vi "Generate Waveform in LV.vi"() -> (3 "a2":T1={"String"="This NULL (\u0000) is inside a LV Cluster", "Boolean"=FALSE, "Array"=[1.0+0.0i, 2.0+0.0i, 3.0+0.0i, 0.0+4.0i, 0.0+5.0i, 0.0+6.0i, 7.0+8.0i, 9.0+10.0i, -1.0-2.0i, -1e+20+1e+36i, 6.023e+23-1.23e-118i]}, 4 "waveform out":waveform(dbl), 6 "t0":timestamp, 8 "dt":dbl, 10 "Y":dbl[](array[numeric]), 15 "a1":string="This is a LabVIEW\nstring with a NULL (\u0000) character inside")   [LabVIEW 2013]
uses:
  <vilib>/measure/NI_MABase.lvlib
panel:
  in  "Cluster":T1={"String"="This NULL (\u0000) is inside a LV Cluster", "Boolean"=FALSE, "Array"=[1.0+0.0i, 2.0+0.0i, 3.0+0.0i, 0.0+4.0i, 0.0+5.0i, 0.0+6.0i, 7.0+8.0i, 9.0+10.0i, -1.0-2.0i, -1e+20+1e+36i, 6.023e+23-1.23e-118i]}
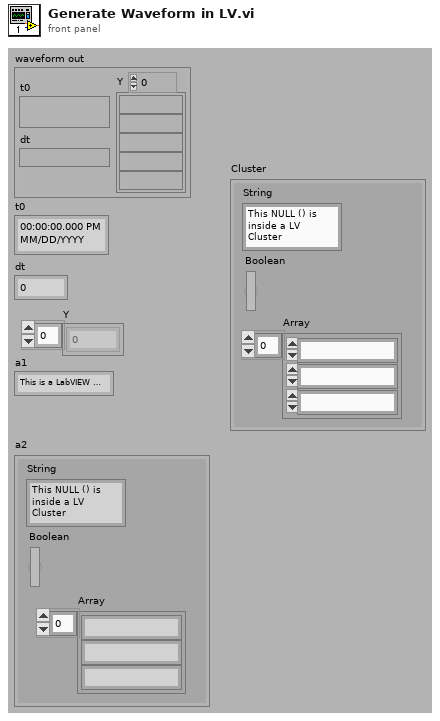
[diagram p1: front panel]
types:
  T1 = cluster{"String":string, "Boolean":bool, "Array":cxt[]}
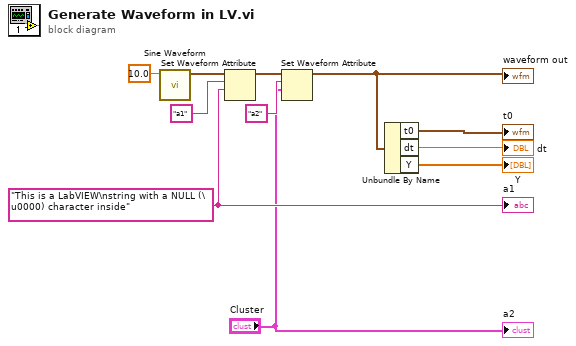
[diagram p0: block diagram]
diagram:
  w5 = "This is a LabVIEW\nstring with a NULL (\u0000) character inside"
  n1 = call <vilib>:"Sine Waveform.vi"("frequency"=10.0) -> ("signal out"=w10:waveform(dbl))  [unwired: 6 in, 4 out]
  n2 = Set Waveform Attribute(5:w5, 6:"a1", 7:w10) -> (3:w4:waveform(dbl))  [unwired: 1 in, 2 out]
  n3 = Set Waveform Attribute(5:"Cluster", 6:"a2" ("name"), 7:w4) -> (3:w3:waveform(dbl))  [unwired: 1 in, 2 out]
  "waveform out" <- w3
  n4 = Unbundle By Name(w3) -> ("t0"=→"t0":timestamp, "dt"=→"dt":dbl, "Y"=→"Y":dbl[])
  "a1" <- w5
  "a2" <- "Cluster"
